vi "Test 2 Get value example 4.vi"(8 "error in (no error)":errorcluster, 11 "Test Case In":refnum<class "Descrambler Test.lvclass">) -> (0 "error out":errorcluster, 3 "Test Case Out":refnum<class "Descrambler Test.lvclass">)   [LabVIEW 2020, in "Descrambler Test.lvclass"]
uses:
  Descrambler Test.lvclass
  Descrambler Test.lvclass/Descrambler Test.ctl
  4993e8ee-a06a-463a-9684-69129f64d5ce.vi
  Descrambler/Descrambler.lvclass
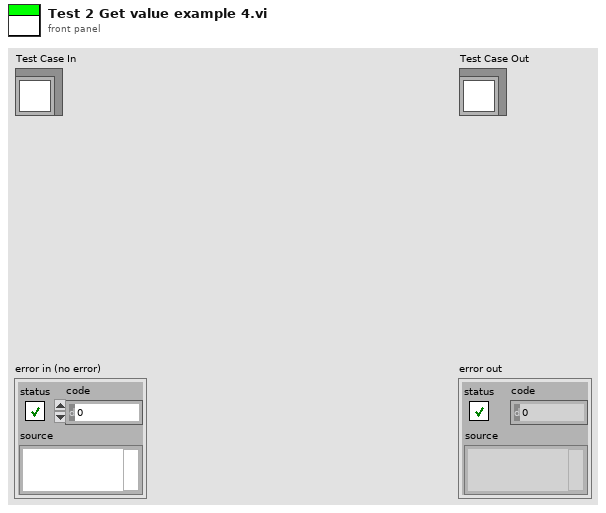
[diagram p1: front panel]
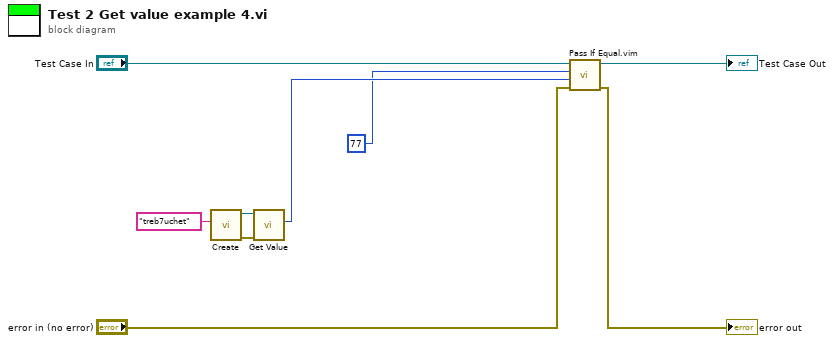
[diagram p0: block diagram]
diagram:
  n1 = call "Create.vi"("String"="treb7uchet") -> ("error out"=w4:errorcluster, "Descrambler"=w5:refnum<class "Descrambler.lvclass">)  [unwired: 9 in]
  n2 = call "Get Value.vi"("error in (no error)"=w4, "Descrambler in"=w5) -> ("Value"=w3:i32)  [unwired: 7 in, 2 out]
  n3 = call "Pass If Equal.vim"("error in (no error)"="error in (no error)", "Actual"=w3, "Expected"=77, "LUnit Test Case In"="Test Case In") -> ("error out"=→"error out":errorcluster, "LUnit Test Case Out"=→"Test Case Out":refnum<class "Descrambler Test.lvclass">)  [unwired: 6 in]
